vi "State1_3.vi"(0 "Start":bool, 1 "Stop":bool, 2 "t":u32, 3 "Nt":u32, 4 "C_table":cluster{"C":bool, "NC":u32}[](array[cluster]), 6 "Reset":bool, 7 "End step":u32=4) -> (12 "N next":u32, 14 "Start":bool, 15 "Stop":bool, 16 "End":bool, 17 "t":u32, 18 "N curr":u32)   [LabVIEW 2019, in "Userlib.lvlib"]
uses:
  Userlib.lvlib
  Trigers/Triggers.lvlib
  Timer Delay/Timers.lvlib
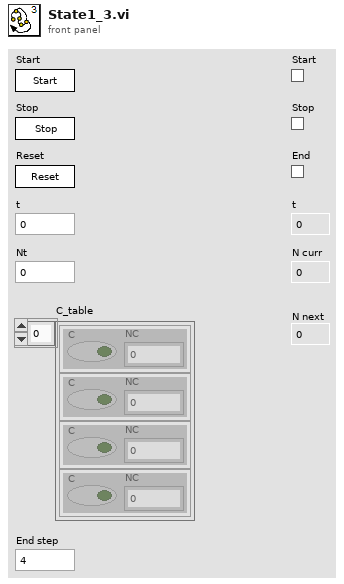
[diagram p1: front panel]
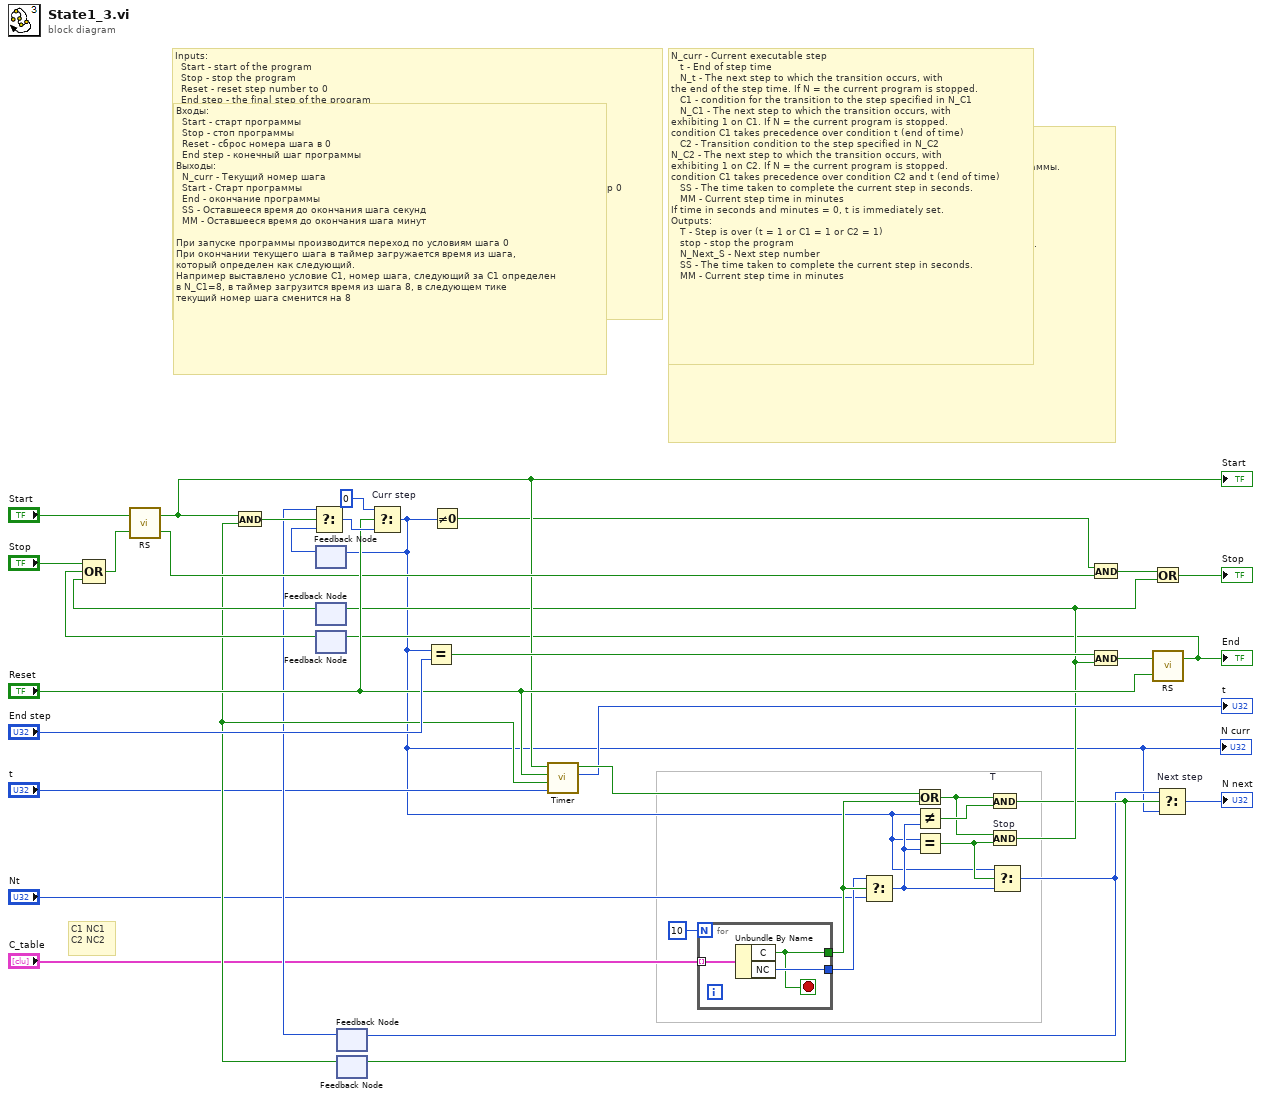
[diagram p0: block diagram]
diagram:
  # "C1 NC1\nC2 NC2"
  # "N_curr - Current executable step\n   t - End of step time\n   N_t - The next step to which the transition occurs, with\nthe end of the step time. If N = the current program is stopped.\n   C1 - condition for the transition to the step specified in N_C1\n   N_C1 - The next step to which the transition occurs, with\nexhibiting 1 on C1. If N = the current program is stopped.\ncondition C1 takes precedence over condition t (end of time)\n   C2 - Transition condition to the step specified in N_C2\nN_C2 - The next step to which the transition occurs, with\nexhibiting 1 on C2. If N = the current program is stopped.\ncondition C1 takes precedence over condition C2 and t (end of time)\n   SS - The time taken to complete the current step in seconds.\n   MM - Current step time in minutes\nIf time in seconds and minutes = 0, t is immediately set.\nOutputs:\n   T - Step is over (t = 1 or C1 = 1 or C2 = 1)\n   stop - stop the program\n   N_Next_S - Next step number\n   SS - The time taken to complete the current step in seconds.\n   MM - Current step time in minutes"
  # "Inputs:\n  Start - start of the program\n  Stop - stop the program\n  Reset - reset step number to 0\n  End step - the final step of the program\nOutputs:\n  N_curr - Current step number\n  Start - Start of the program\n  End - the end of the program\n  SS - Time remaining until the end of the step seconds\n  MM - Time remaining until the end of the step minutes\n\nWhen starting the program, the transition is performed according to the conditions of step 0\nAt the end of the current step, the time from the step is loaded into the timer,\nwhich is defined as the following.\nFor example, condition C1 is set, the step number following C1 is defined\nin N_C1 = 8, the time from step 8 is loaded into the timer, in the next tick\nthe current step number will change to 8"
  # "N_curr - Текущий выполняемый шаг\n  t - Окончание времени шага\n  N_t - Следующий шаг, к которому происходит переход, при\nокончании времени шага. Если N = текущему происходит останов программы.\n  C1 - Условие перехода к шагу, указанному в N_C1\n  N_C1 - Следующий шаг, к которому происходит переход, при\nвыставлении 1 на С1. Если N =текущему происходит останов программы.\nусловие С1 имеет приоритет над условием t (окончание времени)\n  C2 - Условие перехода к шагу, указанному в N_C2\n  N_C2 - Следующий шаг, к которому происходит переход, при\nвыставлении 1 на С2. Если N = текущему происходит останов программы.\nусловие С1 имеет приоритет над условием С2 и t (окончание времени)\n  SS - Время выполнения текущего шага в секундах\n  MM - Время выполнения текущего шага в минутах\nЕсли время в секундах и минутах = 0, сразу выставляется t\nВыходы:\n  T - Шаг окончен (t=1 или C1=1 или С2=1)\n  stop - остановить программу\n  N_Next_S - Номер следующего шага\n  SS - Время выполнения текущего шага в секундах\n  MM - Время выполнения текущего шага в минутах"
  # "Входы:\n  Start - старт программы\n  Stop - стоп программы\n  Reset - сброс номера шага в 0\n  End step - конечный шаг программы\nВыходы:\n  N_curr - Текущий номер шага\n  Start - Старт программы\n  End - окончание программы\n  SS - Оставшееся время до окончания шага секунд\n  MM - Оставшееся время до окончания шага минут\n\nПри запуске программы производится переход по условиям шага 0\nПри окончании текущего шага в таймер загружается время из шага,\nкоторый определен как следующий.\nНапример выставлено условие C1, номер шага, следующий за С1 определен\nв N_C1=8, в таймер загрузится время из шага 8, в следующем тике \nтекущий номер шага сменится на 8"
  n1 = feedback #1() -> (w14:u32)  [unwired: 1 in]
  n2 = feedback #2() -> (w12:bool)  [unwired: 1 in]
  n3 = feedback #3() -> (w10:bool)  [unwired: 1 in]
  n4 = Compound Arithmetic op=OR("Stop", w10, w12) -> (w37:bool)
  n5 = call "RS.vi"("R"=w37, "S"="Start") -> ("~Q"=w22:bool, "Q"=w15:bool)
  "Start" <- w15
  n6 = feedback #4() -> (w6:u32)  [unwired: 1 in]
  n7 = feedback #5() -> (w8:bool)  [unwired: 1 in]
  n8 = And(x=w15, y=w8) -> (x .and. y?=w38:bool)
  n9 = Select(t=w6, s=w38, f=w14) -> (s? t:f=w28:u32)
  n10 = Select "Curr step"(t=u32 0, s="Reset", f=w28) -> (s? t:f=w2:u32)
  "N curr" <- w2
  n11 = feedback-in #1(w2) -> ()
  n12 = Equal?(x=w2, y="End step") -> (x = y?=w25:bool)
  n13 = Not Equal To 0?(x=w2) -> (x != 0?=w1:bool)
  n14 = call "Timer.vi"("ms"="t", "Load (F)"=w8, "Reset (F)"="Reset", "Start (T)"=w15) -> ("t ms"=→"t":u32, "End"=w29:bool)  [unwired: 5 in]
  n15 = for {
    N: 10 -> [_]
    tunnel: "C_table" -> [w41] mode=indexing
    tunnel: [w40] -> w17
    tunnel: [w39] -> w18
    stop <- w39 stop-if-true
    n16 = Unbundle By Name(w41) -> ("C"=w39:bool, "NC"=w40:u32)
  }
  n17 = Select(t=w17, s=w18, f="Nt") -> (s? t:f=w21:u32)
  n18 = Or(x=w29, y=w18) -> (x .or. y?=w31:bool)
  n19 = Not Equal?(x=w2, y=w21) -> (x != y?=w32:bool)
  n20 = Equal?(x=w2, y=w21) -> (x = y?=w30:bool)
  n21 = And "T"(x=w31, y=w32) -> (x .and. y?=w9:bool)
  n22 = feedback-in #5(w9) -> ()
  n23 = And "Stop"(x=w31, y=w30) -> (x .and. y?=w13:bool)
  n24 = feedback-in #2(w13) -> ()
  n25 = Select(t=w2, s=w30, f=w21) -> (s? t:f=w7:u32)
  n26 = feedback-in #4(w7) -> ()
  n27 = And(x=w1, y=w22) -> (x .and. y?=w24:bool)
  n28 = And(x=w25, y=w13) -> (x .and. y?=w34:bool)
  n29 = Or(x=w24, y=w13) -> (x .or. y?=→"Stop":bool)
  n30 = call "RS.vi"("R"="Reset", "S"=w34) -> ("Q"=w11:bool)  [unwired: 1 out]
  "End" <- w11
  n31 = feedback-in #3(w11) -> ()
  n32 = Select "Next step"(t=w7, s=w9, f=w2) -> (s? t:f=→"N next":u32)
